vi "AccumulatedAngle.vi"(11 "Angle In":dbl) -> (3 "Angle Out":dbl)   [LabVIEW 2016]
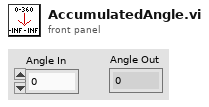
[diagram p1: front panel]
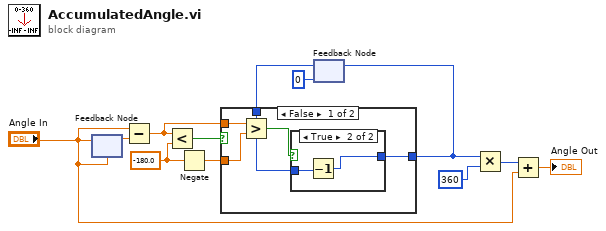
[diagram p0: block diagram]
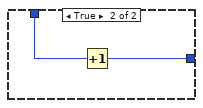
[diagram p3: hidden frame]
diagram:
  w7 = -180.0 ("y")
  n1 = feedback-in #1("Angle In") -> ()
  n2 = feedback #1("Angle In") -> (w12:dbl)
  n3 = Subtract(x="Angle In", y=w12) -> (x-y=w8:dbl)
  n4 = Less?(x=w8, y=w7) -> (x < y?=w11:bool)
  n5 = Negate(x=w7) -> (-x=w6:dbl)
  n6 = feedback #2(0) -> (w9:i32)
  n7 = case shown="False" w11 {
    tunnel: [w13 w22] -> w5
    tunnel: w9 -> [w14 w21]
    tunnel: w8 -> [w17 _]
    tunnel: w6 -> [w16 _]
    frame False {
      n8 = Greater?(x=w17, y=w16) -> (0:w15:bool)
      n9 = case shown="True" w15 {
        tunnel: w14 -> [w18 w20]
        tunnel: [w18 w19] -> w13
        frame False {
        }
        frame True {
          n10 = Decrement(x=w20) -> (x-1=w19:i32)
        }
      }
    }
    frame True {
      n11 = Increment(x=w21) -> (x+1=w22:i32)
    }
  }
  n12 = feedback-in #2(w5) -> ()
  n13 = Multiply(x=w5, y=360) -> (x*y=w3:i32)
  n14 = Add(x=w3, y="Angle In") -> (x+y=→"Angle Out":dbl)
